vi "Open VI Ref.vi"(8 "error in (no error)":errorcluster, 11 "LUnit Test Case In":refnum<class "LUnit Inheriting Test Case.lvclass">) -> (0 "error out":errorcluster, 3 "LUnit Test Case Out":refnum<class "LUnit Inheriting Test Case.lvclass">)   [LabVIEW 2020]
uses:
  LUnit Inheriting Test Case.lvclass
  C:/git/astemes-lunit/source/API/LUnit Test Case/LUnit Test Case.lvclass
  C:/git/astemes-lunit/source/Core/Runnable/Runnable.lvclass
  C:/git/astemes-lunit/source/API/LUnit Inheriting Test Case/LUnit Test Case/LUnit Inheriting Test Case.lvclass
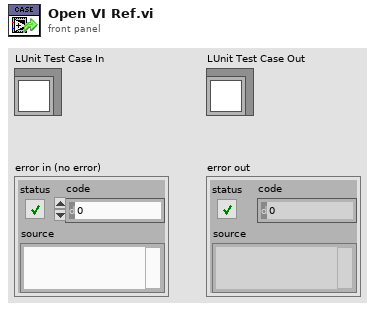
[diagram p1: front panel]
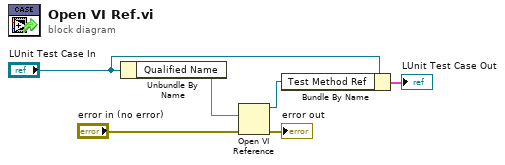
[diagram p0: block diagram]
diagram:
  n1 = Unbundle By Name("LUnit Test Case In") -> ("Qualified Name"=w3)
  n2 = Open VI Reference(vi path=w3, error in (no error)="error in (no error)") -> (vi reference=w1:refnum<vi>, error out=→"error out":errorcluster)  [unwired: 4 in]
  n3 = Bundle By Name(cluster="LUnit Test Case In", "Test Method Ref"=w1) -> (→"LUnit Test Case Out":cluster{})
